vi "CountGlobal.vi"(2 "changed?":bool, 3 "count":i32[](array[numeric])) -> (0 "count out":i32[](array[numeric]))   [LabVIEW 2009]
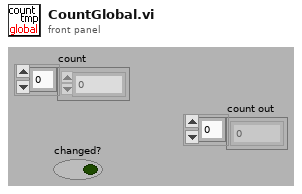
[diagram p1: front panel]
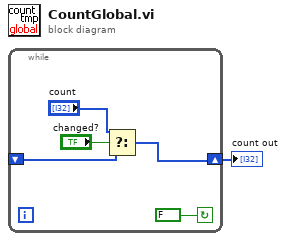
[diagram p0: block diagram]
diagram:
  n1 = while {
    shift-right: [w6] -> w1
    shift-left: _ -> [w4]
    stop <- FALSE continue-if-true
    n2 = Select(t="count", s="changed?", f=w4) -> (s? t:f=w6:i32[])
  }
  "count out" <- w1
